vi "Set Qualified Name.vi"(8 "error in (no error)":errorcluster, 10 "Qualified Name":string, 11 "Test Case in":refnum<class "Test Case.lvclass">) -> (0 "error out":errorcluster, 3 "Test Case out":refnum<class "Test Case.lvclass">)   [LabVIEW 2017, in "Test Case.lvclass"]
uses:
  Test Case.lvclass
  Test Case.lvclass/Test Case.ctl
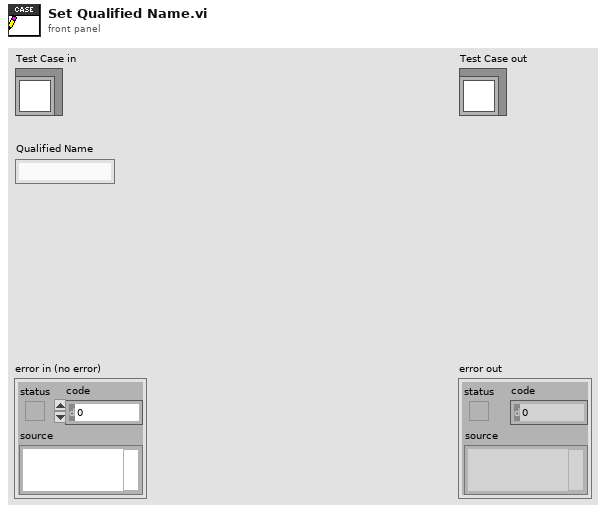
[diagram p1: front panel]
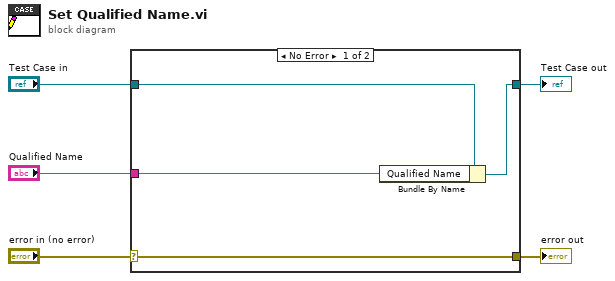
[diagram p0: block diagram]
diagram:
  n1 = case shown="No Error" "error in (no error)" {
    selector: "error in (no error)" -> [w9 w10]
    tunnel: [w9 w10] -> w4
    tunnel: [w7 w11] -> w2
    tunnel: "Test Case in" -> [w8 w11]
    tunnel: "Qualified Name" -> [w6 _]
    frame No Error {
      n2 = Bundle By Name(cluster=w8, "Qualified Name"=w6) -> (w7:refnum<class "Test Case.lvclass">)
    }
    frame Error {
    }
  }
  "error out" <- w4
  "Test Case out" <- w2
